vi "IO_DataQ_WriteDOut.vi"(8 "error in (no error)":errorcluster, 9 "Msg Active":bool, 10 "Message":string[](array[string]), 11 "VISA Refnum in":refnum<visa-resource-name>) -> (0 "error out":errorcluster, 3 "VISA Refnum out":refnum<visa-resource-name>)   [LabVIEW 2024]
doc: "If a Msg Active is true then transmit the Message.."
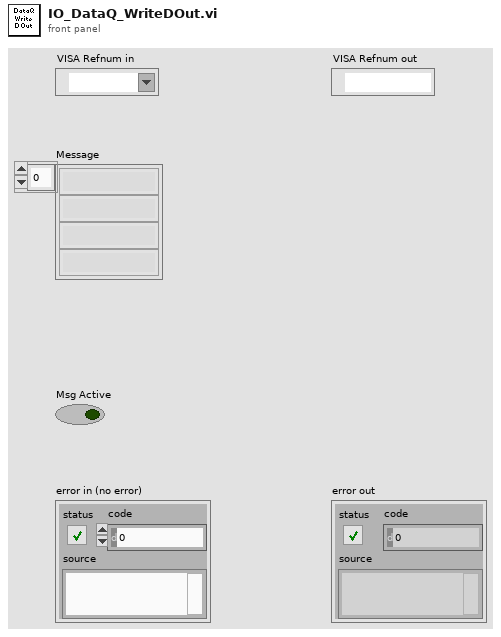
[diagram p1: front panel]
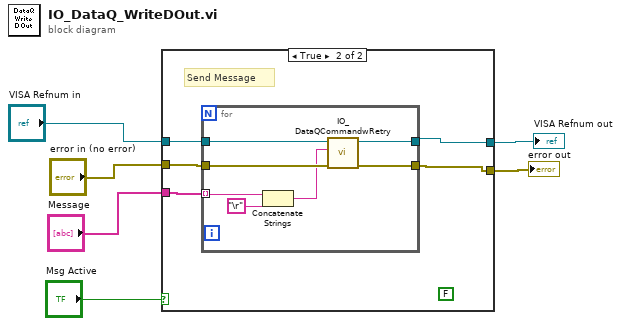
[diagram p0: block diagram]
diagram:
  n1 = case shown="True" "Msg Active" {
    tunnel: [w8 w10] -> w3
    tunnel: [w7 w9] -> w1
    tunnel: "VISA Refnum in" -> [w8 w12]
    tunnel: "error in (no error)" -> [w7 w13]
    tunnel: "Message" -> [_ w11]
    frame False {
      # "Nothing to Send"
    }
    frame True {
      (unwired) FALSE
      # "Send Message"
      n2 = for {
        tunnel: [w18] -> w10
        tunnel: [w17] -> w9
        tunnel: w13 -> [w20]
        tunnel: w12 -> [w19]
        tunnel: w11 -> [w15] mode=indexing
        n3 = Concatenate Strings(w15, "\r") -> (w14:string)
        n4 = call "IO_DataQCommandwRetry.vi"("error in (no error)"=w20, "Command"=w14, "VISA Refnum in"=w19) -> ("error out"=w17:errorcluster, "VISA Refnum out"=w18:refnum<visa-resource-name>)  [unwired: 7 in]
      }
    }
  }
  "error out" <- w1
  "VISA Refnum out" <- w3
